vi "Test Upload.vi"   [LabVIEW 2019]
types:
  T1 = enum16{"open", "replace", "create", "open or create", "replace or create", "replace or create with confirmation"}
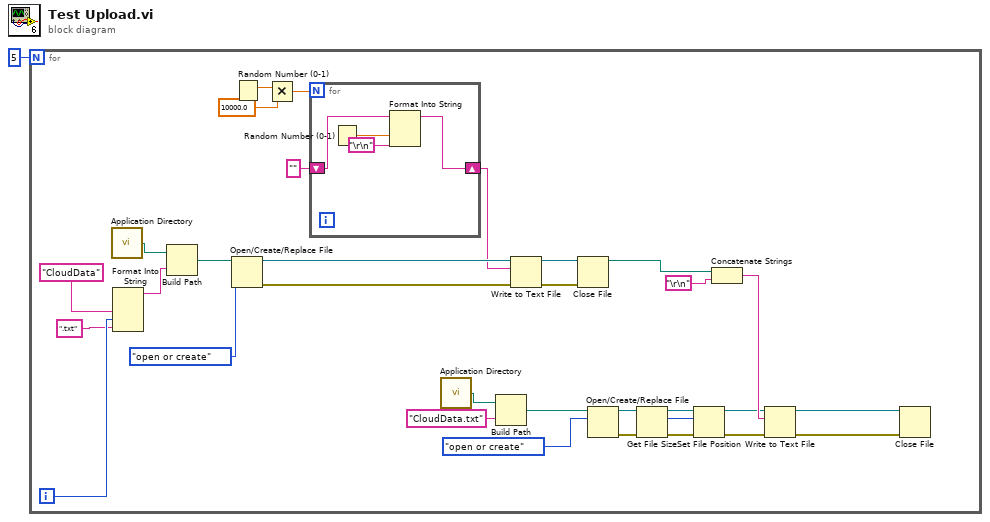
[diagram p0: block diagram]
diagram:
  n1 = for {
    N: 5 -> [_]
    i -> [w13]
    n2 = call <vilib>:"Application Directory.vi"() -> ("Application Directory"=w16:path)
    n3 = Format Into String("CloudData" ("name or relative path"), w13, ".txt" ("name or relative path")) -> (resulting string=w11:string)  [unwired: 3 in, 1 out]
    n4 = Build Path(base path=w16, name or relative path=w11) -> (appended path=w15:path)
    n5 = Open/Create/Replace File(file path (use dialog)=w15, operation (0:open)=T1."open or create") -> (refnum out=w18:refnum<file>, error out=w17:errorcluster)  [unwired: 4 in, 1 out]
    n6 = Random Number (0-1)() -> (number: 0 to 1=w33:dbl)
    n7 = Multiply(x=w33, y=10000.0) -> (x*y=w31:dbl)
    n8 = for {
      N: w31 -> [_]
      shift-right: [w35] -> w9
      shift-left: "" -> [w34]
      n9 = Random Number (0-1)() -> (number: 0 to 1=w37:dbl)
      n10 = Format Into String(initial string=w34, w37, "\r\n") -> (resulting string=w35:string)  [unwired: 2 in, 1 out]
    }
    n11 = call <vilib>:"Application Directory.vi"() -> ("Application Directory"=w24:path)
    n12 = Build Path(base path=w24, name or relative path="CloudData.txt") -> (appended path=w23:path)
    n13 = Write to Text File(file (use dialog)=w18, text=w9, error in=w17) -> (refnum out=w20:refnum<file>, error out=w19:errorcluster)  [unwired: 1 in, 1 out]
    n14 = Close File(refnum=w20, error in=w19) -> (path=w27:path)  [unwired: 1 out]
    n15 = Open/Create/Replace File(file path (use dialog)=w23, operation (0:open)=T1."open or create") -> (refnum out=w8:refnum<file>, error out=w7:errorcluster)  [unwired: 4 in, 1 out]
    n16 = Get File Size(file=w8, error in=w7) -> (refnum out=w4:refnum<file>, size (in bytes)=w6:i64, 0:w5:errorcluster)
    n17 = Set File Position(offset (in bytes) (0)=w6, refnum=w4, error in=w5) -> (refnum out=w3:refnum<file>, error out=w2:errorcluster)  [unwired: 1 in]
    n18 = Concatenate Strings(w27, "\r\n") -> (w25:string)
    n19 = Write to Text File(file (use dialog)=w3, text=w25, error in=w2) -> (refnum out=w29:refnum<file>, error out=w28:errorcluster)  [unwired: 1 in, 1 out]
    n20 = Close File(refnum=w29, error in=w28) -> ()  [unwired: 2 out]
  }
